vi "Rename Recipe In List.vi"(8 "error in (no error)":errorcluster, 9 "New Label":string, 10 "Old Label":string, 11 "ListBox Ref In":refnum<vi>) -> (0 "error out":errorcluster, 2 "Is Valid?":bool, 3 "ListBox Ref Out":refnum<vi>)   [LabVIEW 2021, in "Recipe.lvlib" / "Main Window.lvclass"]
uses:
  Main Window.lvclass
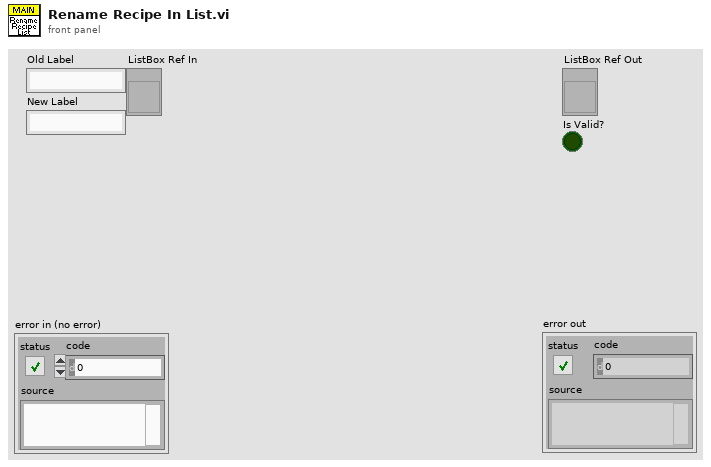
[diagram p1: front panel]
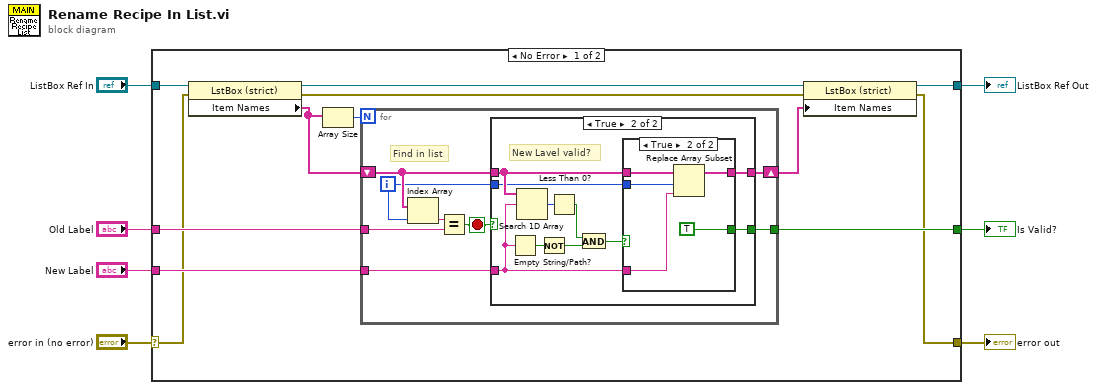
[diagram p0: block diagram]
diagram:
  n1 = case shown="No Error" "error in (no error)" {
    selector: "error in (no error)" -> [w9 w46]
    tunnel: [w14 _] -> w7
    tunnel: "Old Label" -> [w13 _]
    tunnel: "New Label" -> [w12 _]
    tunnel: "ListBox Ref In" -> [w11 w45]
    tunnel: [w10 w45] -> w3
    tunnel: [w8 w46] -> w1
    frame No Error {
      n2 = property class="LstBox (strict)"(reference=w11, error in=w9) -> (reference out=w19:refnum<vi>, error out=w18:errorcluster, "Item Names"=w15:string[])
      n3 = Array Size(array=w15) -> (size(s)=w16:i32)
      n4 = for {
        N: w16 -> [_]
        tunnel: w13 -> [w27]
        tunnel: w12 -> [w26]
        shift-right: [w25] -> w17
        shift-left: w15 -> [w24]
        tunnel: [w20] -> w14
        i -> [w21]
        stop <- w22 stop-if-true
        # "Find in list"
        n5 = Index Array(array=w24, index=w21) -> (element=w23:string)
        n6 = Equal?(x=w23, y=w27) -> (x = y?=w22:bool)
        n7 = case shown="True" w22 {
          tunnel: w26 -> [_ w31]
          tunnel: [w28 w33] -> w25
          tunnel: w24 -> [w28 w34]
          tunnel: w21 -> [_ w30]
          tunnel: [_ w29] -> w20
          frame False {
          }
          frame True {
            # "New Lavel valid?"
            n8 = Empty String/Path?(string/path=w31) -> (empty?=w38:bool)
            n9 = Search 1D Array(1D array=w34, element=w31) -> (index of element=w37:i32)  [unwired: 1 in]
            n10 = Not(x=w38) -> (.not. x?=w35:bool)
            n11 = Less Than 0?(x=w37) -> (x < 0?=w36:bool)
            n12 = And(x=w36, y=w35) -> (x .and. y?=w32:bool)
            n13 = case shown="True" w32 {
              tunnel: w34 -> [w39 w44]
              tunnel: [w39 w43] -> w33
              tunnel: w31 -> [_ w42]
              tunnel: w30 -> [_ w41]
              tunnel: [_ TRUE] -> w29
              frame False {
              }
              frame True {
                n14 = Replace Array Subset(array=w44, new element=w42, index=w41) -> (w43:string[])
              }
            }
          }
        }
      }
      n15 = property class="LstBox (strict)"(reference=w19, error in=w18, "Item Names"=w17) -> (reference out=w10:refnum<vi>, error out=w8:errorcluster)
    }
    frame Error {
    }
  }
  "ListBox Ref Out" <- w3
  "Is Valid?" <- w7
  "error out" <- w1
